vi "0036-Sub_DS18B20.vi"(0 "device":T2, 1 "書き込み":u8[](array[numeric])=[2], 2 "numBytesToWrite":u8=1, 3 "error out":errorcluster) -> (7 "device 2":T2, 8 "数値":dbl, 10 "error out 2":errorcluster caption="error out")   [LabVIEW 2014]
uses:
  <userlib>/LV-CP2112_2014/LVProject/private/CP2112_device.ctl
  <userlib>/LV-CP2112_2014/LVProject/private/CP2112_SMBUS_S0.ctl
panel:
  out "HID_SMBUS_S0":T1
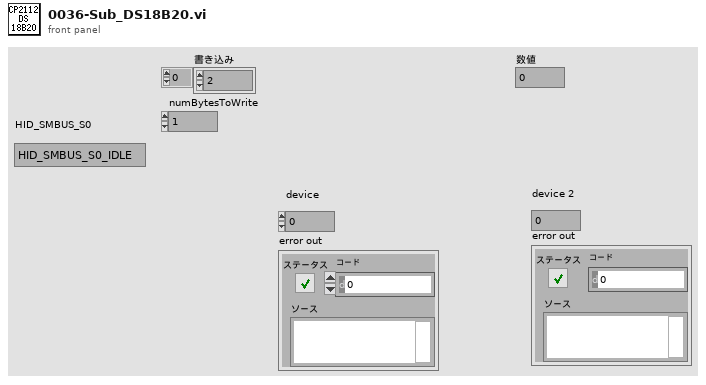
[diagram p1: front panel]
types:
  T1 = typedef "CP2112_SMBUS_S0.ctl" = enum8{"HID_SMBUS_S0_IDLE", "HID_SMBUS_S0_BUSY", "HID_SMBUS_S0_COMPLETE", "HID_SMBUS_S0_ERROR"}
  T2 = typedef "CP2112_device.ctl" = i32
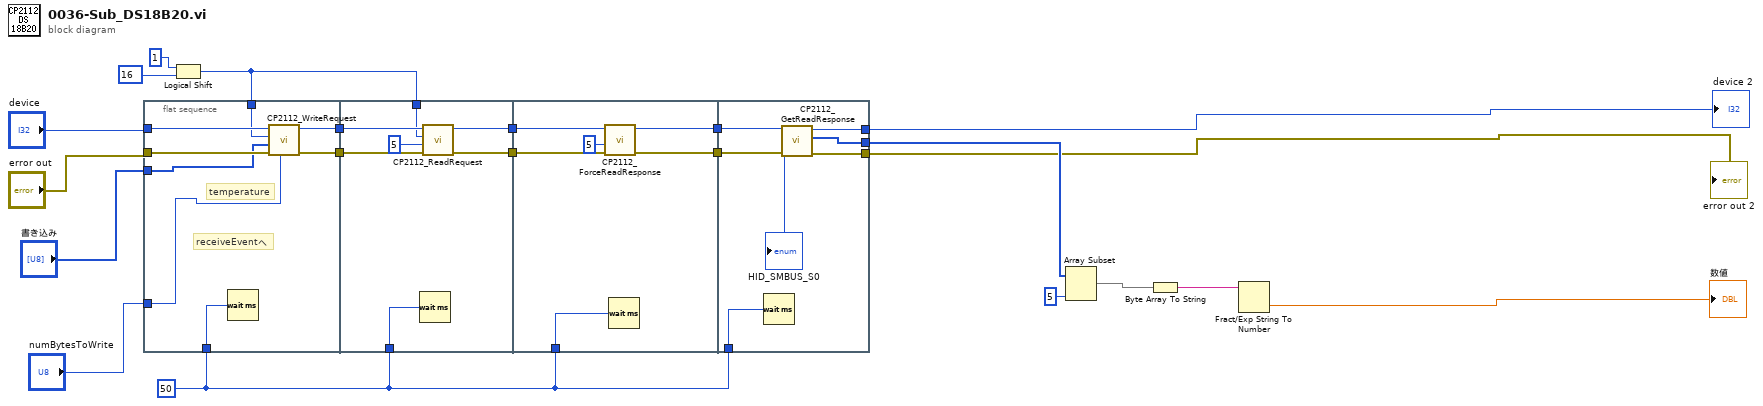
[diagram p0: block diagram]
diagram:
  w6 = u32 50 ("ミリ秒待機時間")
  n1 = flat-sequence {
    tunnel: "device" -> [w29]
    tunnel: "error out" -> [w28]
    tunnel: w12 -> [w25]
    tunnel: [w27] -> w21
    tunnel: [w26] -> w20
    tunnel: w6 -> [w24]
    tunnel: "書き込み" -> [w23]
    tunnel: "numBytesToWrite" -> [w22]
    tunnel: w21 -> [w32]
    tunnel: w20 -> [w33]
    tunnel: w12 -> [w31]
    tunnel: [w35] -> w19
    tunnel: [w34] -> w18
    tunnel: w6 -> [w30]
    tunnel: w19 -> [w40]
    tunnel: w18 -> [w39]
    tunnel: w6 -> [w38]
    tunnel: [w41] -> w17
    tunnel: [w42] -> w16
    tunnel: w17 -> [w45]
    tunnel: w16 -> [w44]
    tunnel: [w48] -> w4
    tunnel: [w47] -> w5
    tunnel: [w46] -> w11
    tunnel: w6 -> [w43]
    frame #0 {
      # "temperature"
      # "receiveEventへ"
      n2 = Wait (ms)(milliseconds to wait=w24) -> ()  [unwired: 1 out]
      n3 = call <userlib>:"CP2112_WriteRequest.vi"("numBytesToWrite"=w22, "error in (no error)"=w28, "buffer"=w23, "slaveAddress"=w25, "device"=w29) -> ("error out"=w27:errorcluster, "deviceOut"=w26:T2)  [unwired: 4 in, 1 out]
    }
    frame #1 {
      n4 = Wait (ms)(milliseconds to wait=w30) -> ()  [unwired: 1 out]
      n5 = call <userlib>:"CP2112_ReadRequest.vi"("error in (no error)"=w32, "numByteToRead"=i16 5, "slaveAddress"=w31, "device"=w33) -> ("error out"=w34:errorcluster, "deviceOut"=w35:T2)  [unwired: 5 in, 1 out]
    }
    frame #2 {
      n6 = call <userlib>:"CP2112_ForceReadResponse.vi"("error in (no error)"=w39, "numByteToRead"=i16 5, "device"=w40) -> ("error out"=w42:errorcluster, "deviceOut"=w41:T2)  [unwired: 6 in, 1 out]
      n7 = Wait (ms)(milliseconds to wait=w38) -> ()  [unwired: 1 out]
    }
    frame #3 {
      n8 = Wait (ms)(milliseconds to wait=w43) -> ()  [unwired: 1 out]
      n9 = call <userlib>:"CP2112_GetReadResponse.vi"("error in (no error)"=w44, "device"=w45) -> ("error out"=w48:errorcluster, "buffer"=w46:u8[], "deviceOut"=w47:T2, "HID_SMBUS_S0"=→"HID_SMBUS_S0":T1)  [unwired: 4 in, 2 out]
    }
  }
  n10 = Logical Shift(y=1, x=16) -> (x << y=w12:i32)
  n11 = Array Subset(array=w11, length=5 ("長さ")) -> (w10:u8[])  [unwired: 1 in]
  n12 = Byte Array To String(unsigned byte array=w10) -> (string=w9:string)
  n13 = Fract/Exp String To Number(string=w9) -> (number=→"数値":dbl)  [unwired: 3 in, 1 out]
  "device 2" <- w5
  "error out 2" <- w4
